vi "Wait2write (SubVI).vi"(11 "millisecond timer value":u32) -> (3 "f":i64)   [LabVIEW 2012]
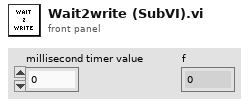
[diagram p1: front panel]
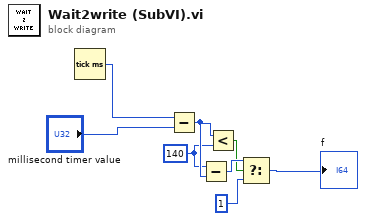
[diagram p0: block diagram]
diagram:
  w3 = i64 140 ("y")
  n1 = Tick Count (ms)() -> (millisecond timer value=w1:u32)
  n2 = Subtract(x=w1, y="millisecond timer value") -> (x-y=w4:u32)
  n3 = Subtract(x=w3, y=w4) -> (x-y=w5:i64)
  n4 = Less?(x=w4, y=w3) -> (x < y?=w2:bool)
  n5 = Select(t=w5, s=w2, f=i64 1) -> (s? t:f=→"f":i64)
